vi "Populate Response Variable.vi"(5 "Variant":variant, 6 "Error in":errorcluster caption="Error in (no error)", 7 "depth":i32, 8 "variable History":string[](array[string]), 9 "String might with variables":string) -> (0 "Error out":errorcluster, 3 "String out":string, 4 "Variant Out":variant)   [LabVIEW 2020]
uses:
  <userlib>/_NEVSTOP/Communicable State Machine(CSM)/addons/INI-Static-Variable-Support/INI-Static-Variable-Support.lvlib
  <userlib>/_NEVSTOP/Communicable State Machine(CSM)/_Shared/CSM Shared.lvlib
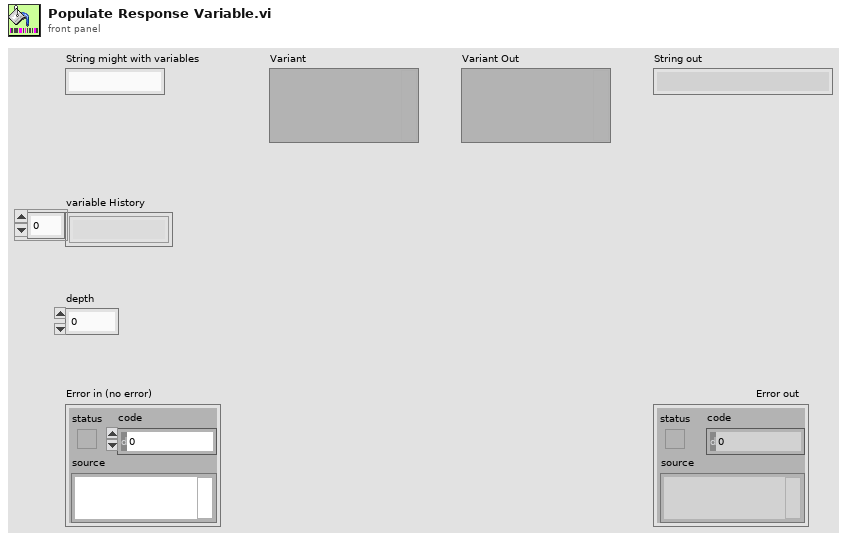
[diagram p1: front panel]
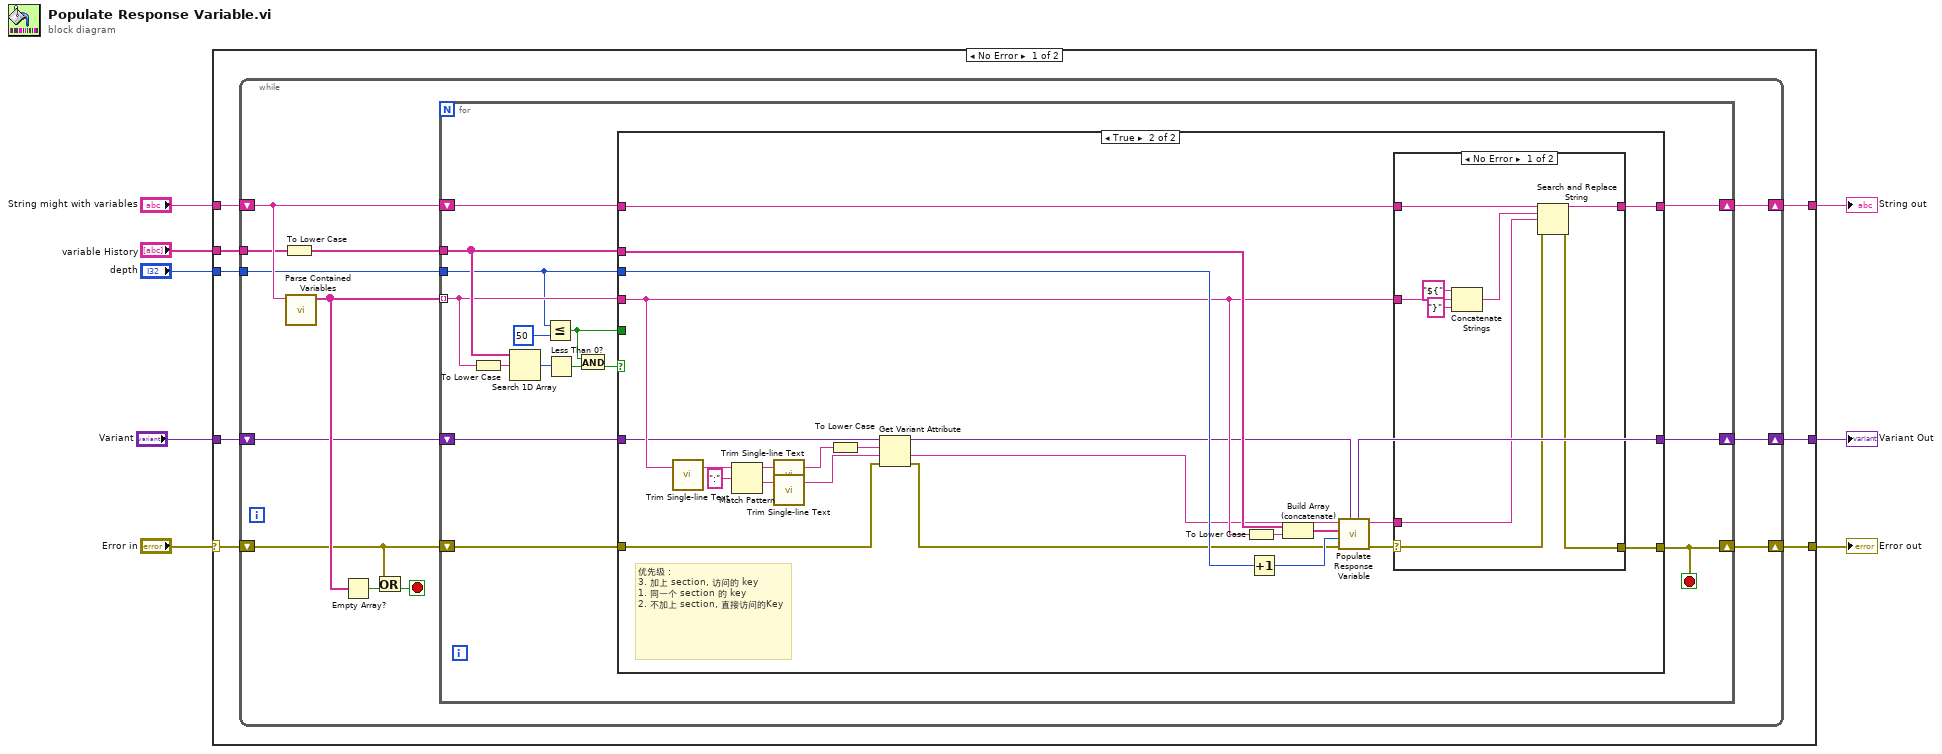
[diagram p0: block diagram]
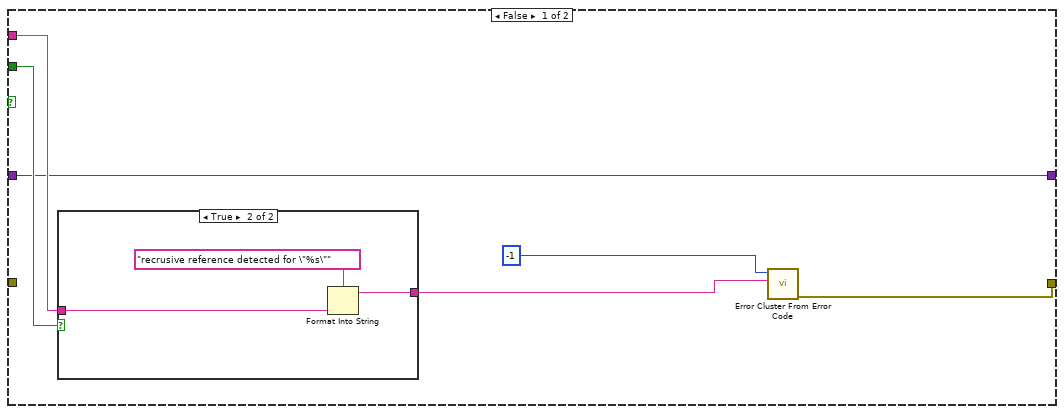
[diagram p2: hidden frame]
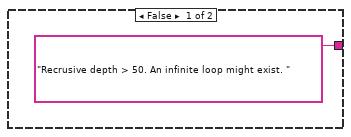
[diagram p3: hidden frame]
diagram:
  n1 = case shown="No Error" "Error in" {
    selector: "Error in" -> [w13 w90]
    tunnel: [w16 w89] -> w8
    tunnel: "String might with variables" -> [w15 w89]
    tunnel: [w12 w90] -> w5
    tunnel: "variable History" -> [w14 _]
    tunnel: "depth" -> [w11 _]
    tunnel: "Variant" -> [w10 w88]
    tunnel: [w9 w88] -> w1
    frame No Error {
      n2 = while {
        shift-right: [w28] -> w16
        shift-left: w15 -> [w26]
        tunnel: w14 -> [w23]
        shift-right: [w24] -> w12
        shift-left: w13 -> [w20]
        tunnel: w11 -> [w19]
        shift-right: [w17] -> w9
        shift-left: w10 -> [w18]
        stop <- w21 stop-if-true
        n3 = To Lower Case(string=w23) -> (all lower case string=w22:string[])
        n4 = call <userlib>:"Parse Contained Variables.vi"("String"=w26) -> ("Contained Variables"=w25:string[])  [unwired: 10 in]
        n5 = Empty Array?(array=w25) -> (empty?=w27:bool)
        n6 = Or(x=w20, y=w27) -> (x .or. y?=w21:bool)
        n7 = for {
          tunnel: w25 -> [w40] mode=indexing
          shift-right: [w42] -> w28
          shift-left: w26 -> [w43]
          tunnel: w22 -> [w41]
          shift-right: [w37] -> w24
          shift-left: w20 -> [w36]
          tunnel: w19 -> [w34]
          shift-right: [w29] -> w17
          shift-left: w18 -> [w30]
          stop <- w37 stop-if-true
          n8 = To Lower Case(string=w40) -> (all lower case string=w39:string)
          n9 = Search 1D Array(1D array=w41, element=w39) -> (index of element=w38:i32)  [unwired: 1 in]
          n10 = Less Or Equal?(x=w34, y=50) -> (x <= y?=w32:bool)
          n11 = Less Than 0?(x=w38) -> (x < 0?=w31:bool)
          n12 = And(x=w32, y=w31) -> (x .and. y?=w35:bool)
          n13 = case shown="True" w35 {
            tunnel: w43 -> [_ w77]
            tunnel: [_ w76] -> w42
            tunnel: [w49 w75] -> w37
            tunnel: w41 -> [_ w65]
            tunnel: w40 -> [w47 w61]
            tunnel: w36 -> [_ w57]
            tunnel: w34 -> [_ w63]
            tunnel: w32 -> [w45 _]
            tunnel: w30 -> [w44 w60]
            tunnel: [w44 w54] -> w29
            frame False {
              n14 = case shown="True" w45 {
                tunnel: w47 -> [_ w52]
                tunnel: ["Recrusive depth > 50. An infinite loop might exist. " w51] -> w46
                frame False {
                }
                frame True {
                  n15 = Format Into String(format string="recrusive reference detected for \"%s\"", w52) -> (resulting string=w51:string)  [unwired: 2 in, 1 out]
                }
              }
              n16 = call <vilib>:"Error Cluster From Error Code.vi"("error message (\"\")"=w46, "error code (0)"=-1 ("code")) -> ("error out"=w49:errorcluster)  [unwired: 7 in]
            }
            frame True {
              # "优先级：\n3. 加上 section, 访问的 key \n1. 同一个 section 的 key\n2. 不加上 section, 直接访问的Key"
              n17 = call <userlib>:"Trim Single-line Text.vi"("single-line text"=w61) -> ("trimed text"=w70:string)  [unwired: 2 in]
              n18 = Match Pattern(string=w70, regular expression=":") -> (before substring=w73:string, after substring=w72:string)  [unwired: 1 in, 2 out]
              n19 = call <userlib>:"Trim Single-line Text.vi"("single-line text"=w73) -> ("trimed text"=w67:string)  [unwired: 2 in]
              n20 = call <userlib>:"Trim Single-line Text.vi"("single-line text"=w72) -> ("trimed text"=w71:string)  [unwired: 2 in]
              n21 = To Lower Case(string=w67) -> (all lower case string=w59:string)
              n22 = Get Variant Attribute(Variant=w60, name=w59, default value (empty Variant)=w71, error in=w57) -> (duplicate Variant=w55:variant, value=w58:string, error out=w56:errorcluster)  [unwired: 1 out]
              n23 = To Lower Case(string=w61) -> (all lower case string=w64:string)
              n24 = Increment(x=w63) -> (x+1=w62:i32)
              n25 = Build Array (concatenate)(w65, w64) -> (w66:string[])
              n26 = call "Populate Response Variable.vi"("Variant"=w55, "Error in"=w56, "depth"=w62, "variable History"=w66, "String might with variables"=w58) -> ("Error out"=w68:errorcluster, "String out"=w69:string, "Variant Out"=w54:variant)  [unwired: 2 in]
              n27 = case shown="No Error" w68 {
                selector: w68 -> [w80 w87]
                tunnel: w77 -> [w84 _]
                tunnel: [w83 _] -> w76
                tunnel: [w82 w87] -> w75
                tunnel: w69 -> [w81 _]
                tunnel: w61 -> [w78 _]
                frame No Error {
                  n28 = Concatenate Strings("${" ("regular expression"), w78, "}" ("regular expression")) -> (w79:string)
                  n29 = Search and Replace String(input string=w84, search string=w79, replace string=w81, error in=w80) -> (result string=w83:string, error out=w82:errorcluster)  [unwired: 4 in, 2 out]
                }
                frame Error {
                }
              }
            }
          }
        }
      }
    }
    frame Error {
    }
  }
  "String out" <- w8
  "Error out" <- w5
  "Variant Out" <- w1
